vi "DronePID1.vi"() -> ()   [LabVIEW 2025]
uses:
  <vilib>/MakerHub/LINX/Public/Peripherals/Analog/Analog Read N Chans.vi
  <vilib>/MakerHub/LINX/Public/Peripherals/PWM/PWM Set Duty Cycle 1 Chan.vi
  <vilib>/MakerHub/LINX/Private/Local IO/LinxAnalogRead.vi
  <vilib>/MakerHub/LINX/Public/Utilities/Check Channel.vi
  <vilib>/MakerHub/LINX/Public/Utilities/Open Serial.vi
  <vilib>/addons/control/pid/pid.llb/PID (DBL).vi
  <vilib>/MakerHub/LINX/Private/Utilties/Generate Error.vi
  <vilib>/MakerHub/LINX/Public/Peripherals/PWM/PWM Set Duty Cycle N Chans.vi
  <vilib>/MakerHub/LINX/LMH-LINX.lvlib
  <vilib>/addons/control/pid/NI_PID_pid.lvlib
panel:
  out "Posicion(Voltaje)":dbl
  in  "PID Gain":T1
  in  "Position":dbl(knob) scale=1.6..3.5
  out "PWM":dbl(graph)
  out "Rotacion":dbl(graph)
  in  "stop":bool
  in  "Serial Port":refnum<visa-resource-name>="N/A"
  # "Tabla Valores\n1,75 V --> -45°\n2,55 V --> 0°\n3,20 V --> 45°"
  # "Valores PID\nKp = 1,2\nKi = 0,04\nKd = 0,003"
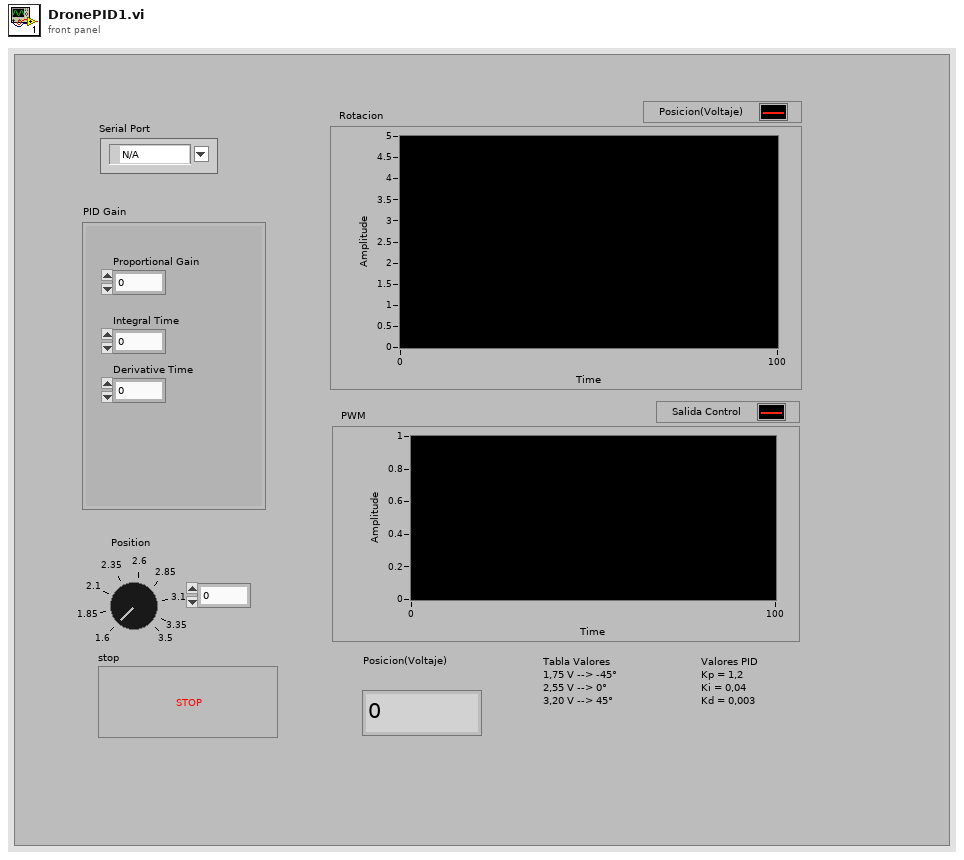
[diagram p1: front panel]
types:
  T1 = cluster{"Proportional Gain":dbl, "Integral Time":dbl, "Derivative Time":dbl}
  T2 = typedef "LMH-LINX.lvlib/LINX Ref.ctl" = cluster{"IO":T3, "Interface":T4, "LINX Device Config":T5}
  T3 = typedef "LMH-LINX.lvlib/Platform.ctl" = enum16{"Remote", "Local"}
  T4 = typedef "LMH-LINX.lvlib/Interface.ctl" = enum16{"Serial", "TCP"}
  T5 = typedef "LMH-LINX.lvlib/Device.lvlib/LINX Device Config.ctl" = cluster{"Interface":T4, "COM Port":refnum<visa-resource-name>, "TCP Configuration":T6, "Device Family":u8, "Device ID":u8, "Device Name":string, "TCP Ref":refnum<k5>, "Channels":T7}
  T6 = typedef "LMH-LINX.lvlib/Device.lvlib/TCP Config.ctl" = cluster{"IP Address":string, "Port":u16}
  T7 = typedef "LMH-LINX.lvlib/Channels.ctl" = cluster{"DI":u8[], "DO":u8[], "AI":u8[], "AO":u8[], "PWM":u8[], "QE":u8[], "UART":u8[], "I2C 2":u8[], "SPI":u8[], "CAN":u8[], "Servo":u8[], "AI Ref (V)":dbl, "AI Resolution (Bits)":u8, "AO Ref (V)":dbl, "AO Resolution (Bits)":u8}
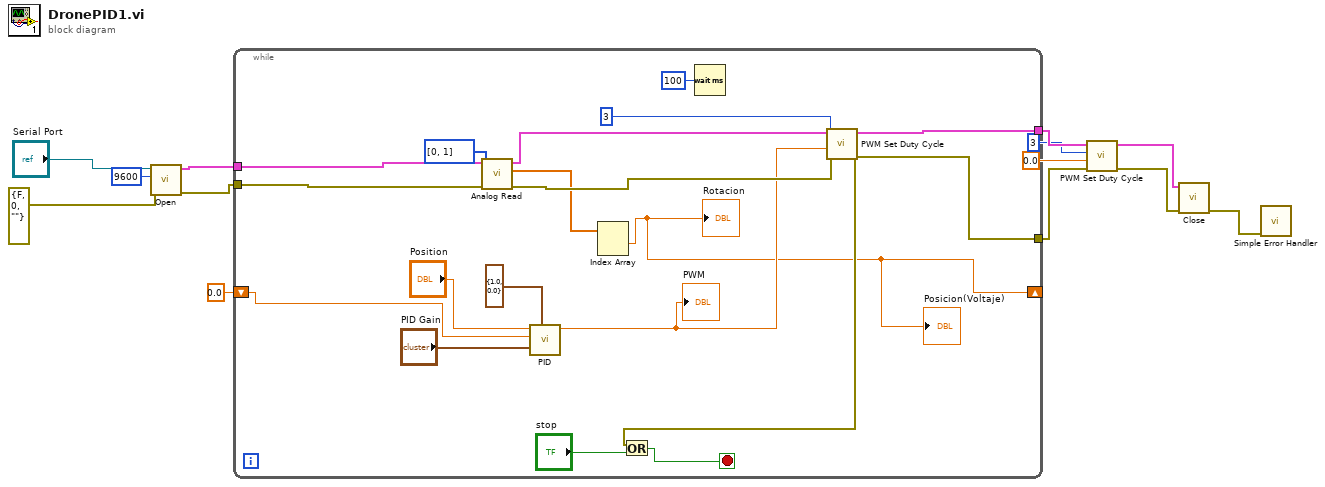
[diagram p0: block diagram]
diagram:
  n1 = call-poly <vilib>:"Open.vi"("Error In"=errorcluster {"status"=FALSE, "code"=0, "source"=""}, "Baud Rate Override"=u32 9600, "Serial Port"="Serial Port") -> ("Error Out"=w9:errorcluster, "LINX Resource"=w10:T2)  [unwired: 6 in, 1 out]
  n2 = while {
    tunnel: w10 -> [w31]
    tunnel: w9 -> [w30]
    tunnel: [w21] -> w3
    tunnel: [w20] -> w6
    shift-right: [w14] -> _
    shift-left: 0.0 ("Numeric Control") -> [w16]
    stop <- w24 stop-if-true
    n3 = call-poly <vilib>:"Analog Read.vi"("Error In"=w30, "AI Channel(s)"=u8[] [0, 1], "LINX Resource"=w31) -> ("Error Out"=w26:errorcluster, "Voltages"=w22:dbl[], "LINX Resource"=w29:T2)  [unwired: 5 in, 1 out]
    n4 = call-poly <vilib>:"PID.vi"("output range"=cluster{"output high":dbl, "output low":dbl} {"output high"=1.0, "output low"=0.0}, "PID gains"="PID Gain", "process variable"=w16, "setpoint"="Position") -> ("output"=w15:dbl)  [unwired: 6 in, 1 out]
    "PWM" <- w15
    n5 = Index Array(array=w22) -> (element #1=w14:dbl)  [unwired: 2 in, 1 out]
    "Rotacion" <- w14
    "Posicion(Voltaje)" <- w14
    n6 = Wait (ms)(milliseconds to wait=u32 100) -> ()  [unwired: 1 out]
    n7 = call-poly <vilib>:"PWM Set Duty Cycle.vi"("Error In"=w26, "Duty Cycle (0-1)"=w15, "PWM Channel"=u8 3, "LINX Resource"=w29) -> ("Error Out"=w21:errorcluster, "LINX Resource"=w20:T2)  [unwired: 6 in]
    n8 = Or(x=w21, y="stop") -> (x .or. y?=w24:bool)
  }
  n9 = call-poly <vilib>:"PWM Set Duty Cycle.vi"("Error In"=w3, "Duty Cycle (0-1)"=0.0, "PWM Channel"=u8 3, "LINX Resource"=w6) -> ("Error Out"=w2:errorcluster, "LINX Resource"=w1:T2)  [unwired: 6 in]
  n10 = call <vilib>:"Close.vi"("Error In"=w2, "LINX Resource"=w1) -> ("Error Out"=w8:errorcluster)  [unwired: 9 in]
  n11 = call <vilib>:"Simple Error Handler.vi"("error in (no error)"=w8) -> ()  [unwired: 4 in, 5 out]
